vi "ParseChanProps.vi"(11 "properties":T3[](array[typedef])) -> (1 "invalid":bool, 3 "channel":T1)   [LabVIEW 2017, in "ModbusMaster.lvlib"]
uses:
  <vilib>/addons/InsightCM/Devices/Shared/Common/ModbusMaster/ModbusMaster.lvlib
  <vilib>/addons/InsightCM/MessageBus/Base/controls/KeyValuePair.ctl
  <vilib>/addons/InsightCM/Devices/Shared/Common/ModbusMaster/controls/ModbusChannel.ctl
  <vilib>/addons/InsightCM/Devices/Shared/Common/ModbusMaster/controls/RegisterType.ctl
  <vilib>/addons/InsightCM/Utilities/PropertyHelpers/PropertyHelpers.lvlib
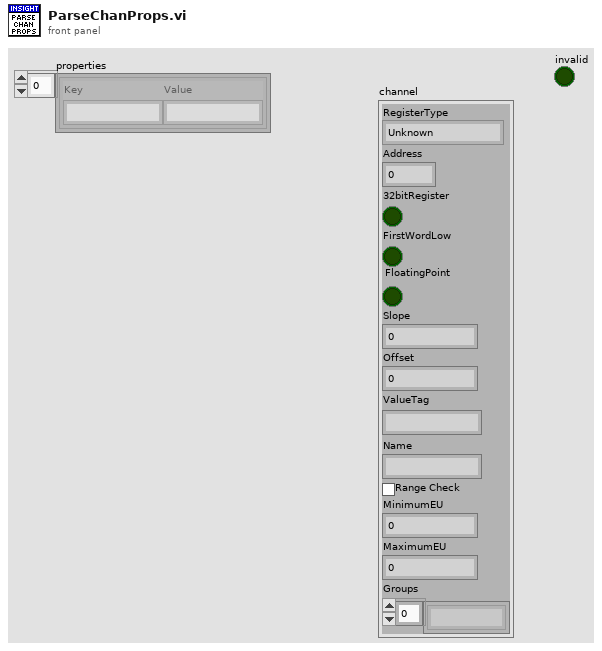
[diagram p1: front panel]
types:
  T1 = typedef "ModbusMaster.lvlib/ModbusChannel.ctl" = cluster{"RegisterType":T2, "Address":i32, "32bitRegister":bool, "FirstWordLow":bool, "FloatingPoint":bool, "Slope":dbl, "Offset":dbl, "ValueTag":string, "Name":string, "Range Check":bool, "MinimumEU":dbl, "MaximumEU":dbl, "Groups":string[]}
  T2 = typedef "ModbusMaster.lvlib/RegisterType.ctl" = enum16{"Unknown", "Coil", "Discrete Input", "Holding Register", "Input Register"}
  T3 = typedef "KeyValuePair.ctl" = cluster{"Key":string, "Value":string}
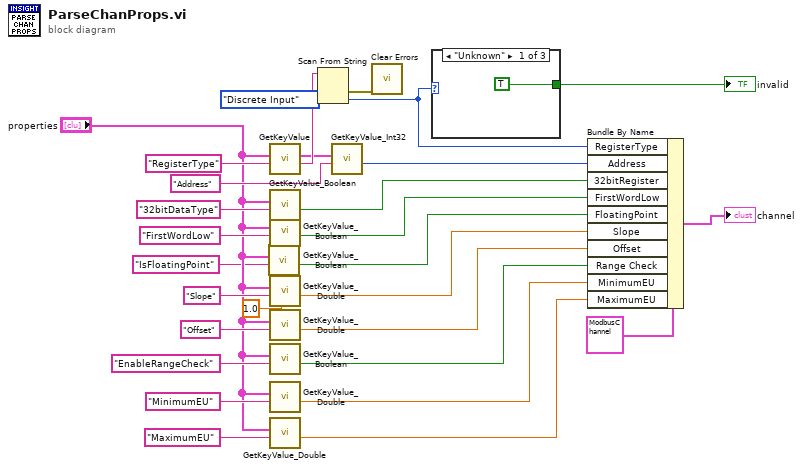
[diagram p0: block diagram]
diagram:
  n1 = call <vilib>:"GetKeyValue_Boolean.vi"("key"="IsFloatingPoint", "key value pairs"="properties") -> ("value"=w1:bool)  [unwired: 7 in, 2 out]
  n2 = call <vilib>:"GetKeyValue.vi"("key"="RegisterType", "key value pairs"="properties") -> ("value"=w27:string, "key value pairs out"=w24:T3[])  [unwired: 7 in, 1 out]
  n3 = call <vilib>:"GetKeyValue_Boolean.vi"("key"="32bitDataType", "key value pairs"="properties") -> ("value"=w21:bool)  [unwired: 7 in, 2 out]
  n4 = call <vilib>:"GetKeyValue_Boolean.vi"("key"="FirstWordLow", "key value pairs"="properties") -> ("value"=w18:bool)  [unwired: 7 in, 2 out]
  n5 = call <vilib>:"GetKeyValue_Double.vi"("default"=1.0, "key"="Slope", "key value pairs"="properties") -> ("value"=w2:dbl)  [unwired: 6 in, 2 out]
  n6 = call <vilib>:"GetKeyValue_Double.vi"("key"="Offset", "key value pairs"="properties") -> ("value"=w11:dbl)  [unwired: 7 in, 2 out]
  n7 = call <vilib>:"GetKeyValue_Boolean.vi"("key"="EnableRangeCheck", "key value pairs"="properties") -> ("value"=w7:bool)  [unwired: 7 in, 2 out]
  n8 = call <vilib>:"GetKeyValue_Double.vi"("key"="MinimumEU", "key value pairs"="properties") -> ("value"=w6:dbl)  [unwired: 7 in, 2 out]
  n9 = call <vilib>:"GetKeyValue_Double.vi"("key"="MaximumEU", "key value pairs"="properties") -> ("value"=w5:dbl)  [unwired: 7 in, 2 out]
  n10 = Scan From String(input string=w27, default 1=RegisterType."Discrete Input" ("RegisterType")) -> (error out=w26:errorcluster, output 1=w17:T2)  [unwired: 3 in, 2 out]
  n11 = call <vilib>:"GetKeyValue_Int32.vi"("key"="Address", "key value pairs"=w24) -> ("value"=w22:i32)  [unwired: 7 in, 2 out]
  n12 = call <vilib>:"Clear Errors.vi"("error in (no error)"=w26) -> ()  [unwired: 5 in, 2 out]
  n13 = case shown="\"Unknown\"" w17 {
    tunnel: [TRUE _ _] -> w16
    frame "Unknown" {
    }
    frame "Coil", "Discrete Input" {
    }
    frame "Holding Register", "Input Register" {
    }
  }
  "invalid" <- w16
  n14 = Bundle By Name(cluster=T1 {"RegisterType"=enum."Unknown", "Address"=0, "32bitRegister"=FALSE, "FirstWordLow"=FALSE, "FloatingPoint"=FALSE, "Slope"=0.0, "Offset"=0.0, "ValueTag"="", "Name"="", "Range Check"=FALSE, "MinimumEU"=0.0, "MaximumEU"=0.0, "Groups"=[]} ("channel"), "RegisterType"=w17, "Address"=w22, "32bitRegister"=w21, "FirstWordLow"=w18, "FloatingPoint"=w1, "Slope"=w2, "Offset"=w11, "Range Check"=w7, "MinimumEU"=w6, "MaximumEU"=w5) -> (→"channel":T1)
